vi "dynamatic.vi"(8 "error in (no error)":errorcluster, 11 "IBar in":refnum<class "IBar.lvclass">) -> (0 "error out":errorcluster, 3 "IBar out":refnum<class "IBar.lvclass">)   [LabVIEW 2021, in "IBar.lvclass"]
uses:
  IBar.lvclass
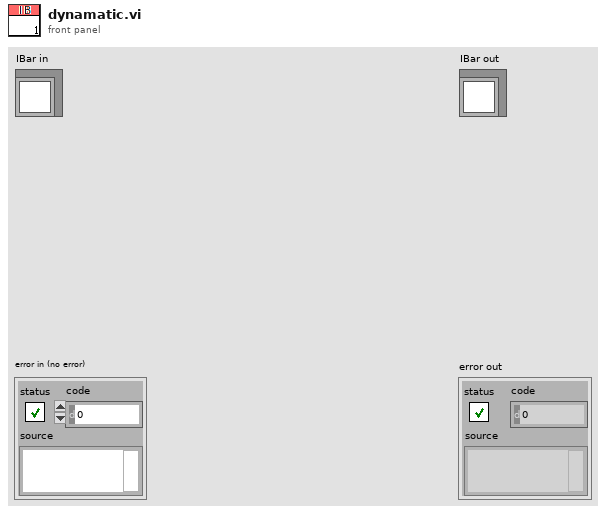
[diagram p1: front panel]
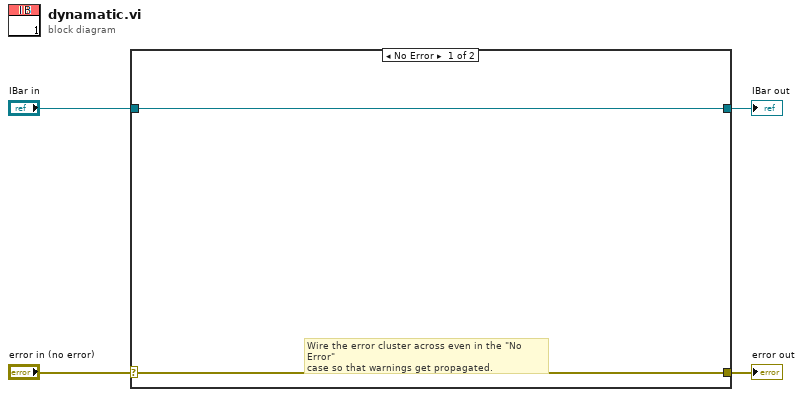
[diagram p0: block diagram]
diagram:
  n1 = case shown="No Error" "error in (no error)" {
    selector: "error in (no error)" -> [w5 w8]
    tunnel: [w5 w8] -> w3
    tunnel: [w6 w7] -> w1
    tunnel: "IBar in" -> [w6 w7]
    frame No Error {
      # "Wire the error cluster across even in the \"No Error\"\ncase so that warnings get propagated."
    }
    frame Error {
    }
  }
  "error out" <- w3
  "IBar out" <- w1
